vi "AMC e.bloxx Initialize.vi"(6 "stop bits (10: 1 bit)":u16(ring)=10 items=["1.0"=10, "1.5"=15, "2.0"=20], 7 "parity (0:none)":enum16{"None", "Odd", "Even", "Mark", "Space"}(ring), 8 "error in (no error)":errorcluster, 9 "data bits (8)":u16=8 min=5 max=8 step=1, 10 "baud rate (9600)":u32=9600, 11 "VISA resource name":refnum<visa-resource-name>) -> (0 "error out":errorcluster, 3 "VISA resource name out":refnum<visa-resource-name>)   [LabVIEW 2013]
doc: "<B>AMC - Analytik & Messtechnik GmbH Chemnitz</B>\n\nLabVIEW Drivers for e.bloxx series from Gantner Instruments\n\nThis VI initializes and opens the serial port specified by <B>VISA resource name</B>."
uses:
  <vilib>/Instr/_visa.llb/VISA Configure Serial Port (Instr).vi
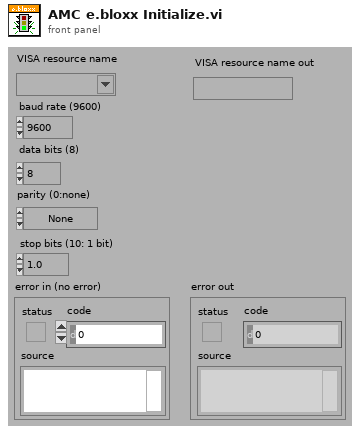
[diagram p1: front panel]
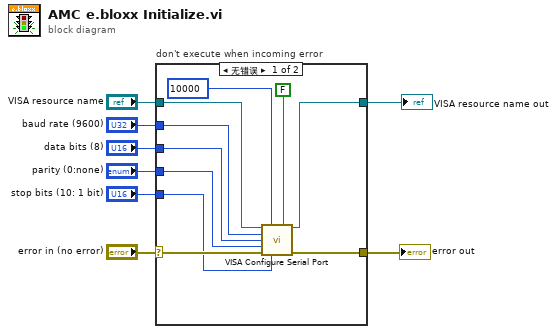
[diagram p0: block diagram]
diagram:
  n1 = case "don't execute when incoming error" shown="无错误" "error in (no error)" {
    selector: "error in (no error)" -> [w18 w20]
    tunnel: [w17 w20] -> w7
    tunnel: "VISA resource name" -> [w16 w19]
    tunnel: "baud rate (9600)" -> [w15 _]
    tunnel: "data bits (8)" -> [w14 _]
    tunnel: "parity (0:none)" -> [w13 _]
    tunnel: "stop bits (10: 1 bit)" -> [w12 _]
    tunnel: [w11 w19] -> w1
    frame No Error {
      n2 = call-poly "VISA Configure Serial Port"("VISA resource name"=w16, "timeout (10sec)"=u32 10000, "Enable Termination\nChar (T)"=FALSE ("Enable Termination\nChar (T)"), "baud rate (9600)"=w15, "data bits (8)"=w14, "parity (0:none)"=w13, "error in (no error)"=w18, "stop bits (10: 1 bit)"=w12) -> ("VISA resource name out"=w11:refnum<visa-resource-name>, "error out"=w17:errorcluster)  [unwired: 6 in]
    }
    frame Error {
    }
  }
  "error out" <- w7
  "VISA resource name out" <- w1
